vi "MVE FXP TD.vi"(11 "showOverflowBit?":i32) -> (2 "typeDescriptor":u8[](array[numeric]), 3 "Cancelled":bool)   [LabVIEW 2016]
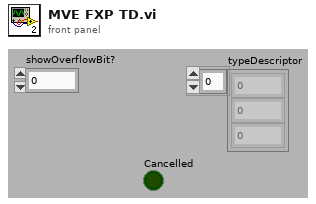
[diagram p1: front panel]
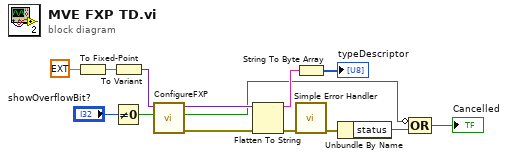
[diagram p0: block diagram]
diagram:
  n1 = To Fixed-Point(number=ext 0.0) -> (fixed-point=w5:fxp<+/-,32,16>)  [unwired: 1 in]
  n2 = Not Equal To 0?(x="showOverflowBit?") -> (x != 0?=w1:bool)
  n3 = To Variant(anything=w5) -> (Variant=w3:variant)
  n4 = call <vilib>:"ConfigureFXP.vi"("show include overflow status?"=w1, "variant in"=w3) -> ("error out"=w9:errorcluster, "changed?"=w11:bool, "variant out"=w12:variant)  [unwired: 7 in]
  n5 = Flatten To String(anything=w12, error in (no error)=w9) -> (data string=w13:string, error out=w7:errorcluster)  [unwired: 2 in, 1 out]
  n6 = String To Byte Array(string=w13) -> (unsigned byte array=→"typeDescriptor":u8[])
  n7 = call <vilib>:"Simple Error Handler.vi"("error in (no error)"=w7) -> ("error out"=w6:errorcluster)  [unwired: 4 in, 4 out]
  n8 = Unbundle By Name(w6) -> ("status"=w8:bool)
  n9 = Compound Arithmetic op=OR(invert w11, w8) -> (→"Cancelled":bool)
